vi "Set Occurrence.vi"(7 "occurrence":refnum<k4>, 8 "error in (no error)":errorcluster, 11 "Valve in":refnum<class "Valve.lvclass">) -> (0 "error out":errorcluster, 3 "Valve out":refnum<class "Valve.lvclass">)   [LabVIEW 2015, in "cRIO-Carbondioxide.lvlib" / "CO2-Actor.lvlib" / "Valve.lvclass"]
uses:
  Valve.lvclass
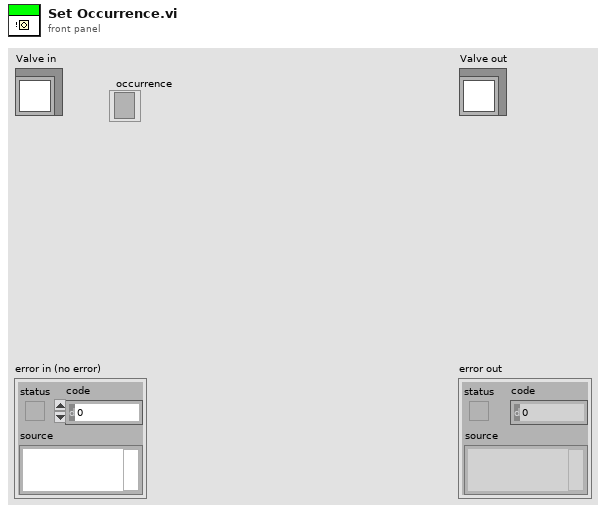
[diagram p1: front panel]
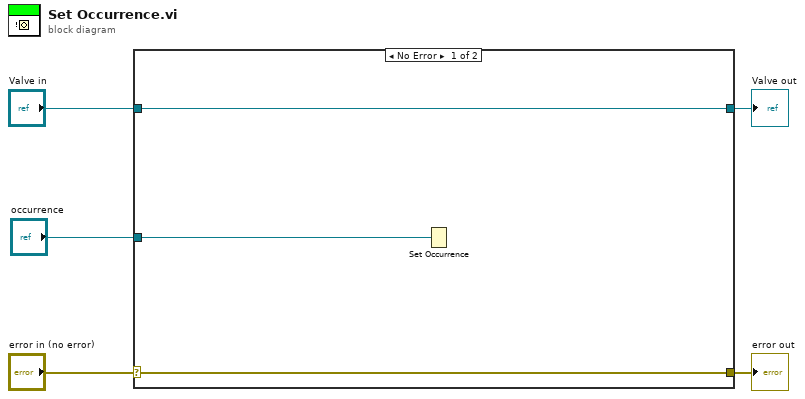
[diagram p0: block diagram]
diagram:
  n1 = case shown="No Error" "error in (no error)" {
    selector: "error in (no error)" -> [w7 w10]
    tunnel: [w7 w10] -> w4
    tunnel: [w8 w9] -> w2
    tunnel: "Valve in" -> [w8 w9]
    tunnel: "occurrence" -> [w6 _]
    frame No Error {
      n2 = Set Occurrence(w6) -> ()
    }
    frame Error {
    }
  }
  "error out" <- w4
  "Valve out" <- w2
